vi "Audio_transformation_v001.vi"() -> ()   [LabVIEW 2019]
uses:
  <vilib>/sound2/lvsound2.llb/Sound Data Format.ctl
  <vilib>/sound2/lvsound2.llb/Sound Input Read (DBL).vi
  <vilib>/addons/Time Frequency Analysis/Transform.llb/TFA Online Gabor Transform (Real).vi
  <vilib>/addons/_Advanced Signal Processing/NI_AdvSigProcTFA.lvlib
panel:
  out "Magnitude of Gabor Coefficients":dbl[][](graph)
  out "Noise Speech":dbl[](graph)
  in  "stop":bool
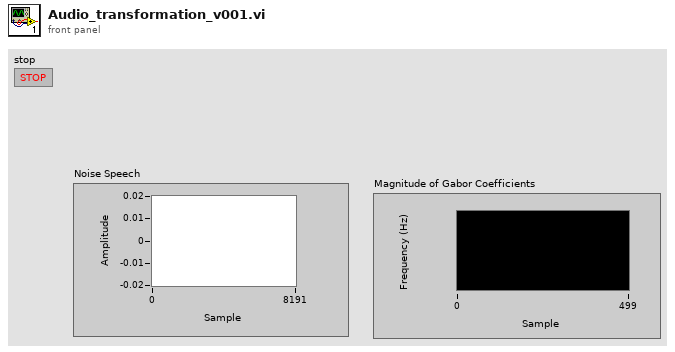
[diagram p1: front panel]
types:
  T1 = typedef "Sound Data Format.ctl" = cluster{"sample rate (S/s)":dbl, "number of channels":i32, "bits per sample":i32}
  T2 = typedef "Sound Input Task ID.ctl" = u32
  T3 = cluster{"analysis window":dbl[], "dM (time steps)":i32, "N (frequency bins)":i32}
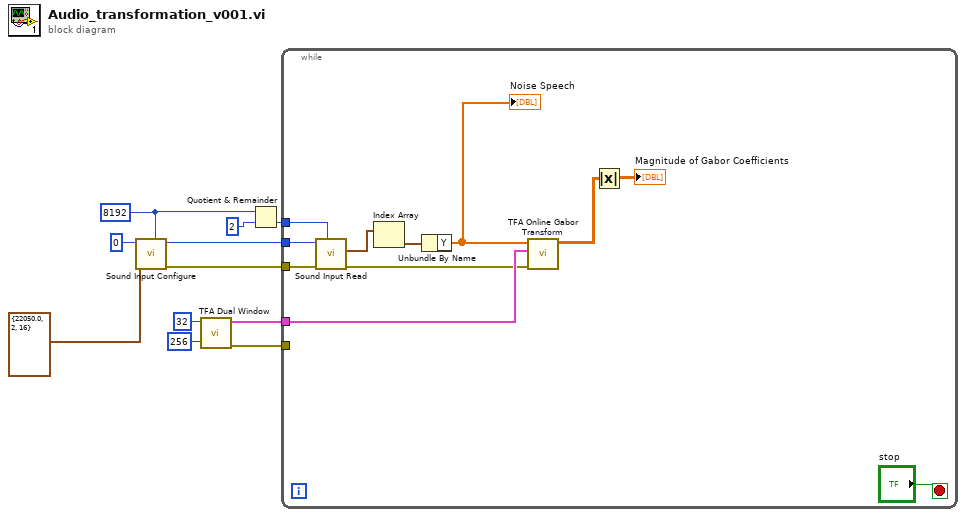
[diagram p0: block diagram]
diagram:
  w8 = 8192 ("number of samples/ch")
  n1 = call <vilib>:"Sound Input Configure.vi"("number of samples/ch"=w8, "sound format"=T1 {"sample rate (S/s)"=22050.0, "number of channels"=2, "bits per sample"=16}, "device ID"=u32 0) -> ("error out"=w5:errorcluster, "task ID"=w9:T2)  [unwired: 7 in]
  n2 = call <vilib>:"TFA Dual Window.vi"("N (frequency bins)"=256, "dM (time steps)"=32) -> ("error out"=w2:errorcluster, "analysis info"=w1:T3)  [unwired: 7 in, 1 out]
  n3 = Quotient & Remainder(x=w8, y=2) -> (floor(x/y)=w6:i32)  [unwired: 1 out]
  n4 = while {
    tunnel: w9 -> [w21]
    tunnel: w6 -> [w20]
    tunnel: w5 -> [w19]
    tunnel: w2 -> [_]
    tunnel: w1 -> [w16]
    stop <- "stop" stop-if-true
    n5 = call-poly <vilib>:"Sound Input Read.vi"("number of samples/ch"=w20, "error in (no error)"=w19, "task ID"=w21) -> ("error out"=w15:errorcluster, "data"=w18:waveform(dbl)[])  [unwired: 6 in, 1 out]
    n6 = Index Array(array=w18) -> (element=w17:waveform(dbl))  [unwired: 1 in]
    n7 = Unbundle By Name(w17) -> ("Y"=w13:dbl[])
    "Noise Speech" <- w13
    n8 = call-poly <vilib>:"TFA Online Gabor Transform.vi"("error in (no error)"=w15, "transform info"=w16, "signal"=w13) -> ("Gabor coef"=w14:cdb[][])  [unwired: 6 in, 2 out]
    n9 = Absolute Value(x=w14) -> (abs(x)=→"Magnitude of Gabor Coefficients":dbl[][])
  }
